vi "Com_Panel_Panel Fit Origin.vi"(8 "error in":errorcluster, 11 "VI Refnum In":refnum<vi>) -> (0 "error out":errorcluster, 3 "VI Refnum Out":refnum<vi>)   [LabVIEW 2016]
uses:
  <vilib>/Utility/miscctls.llb/LVPointTypeDef.ctl
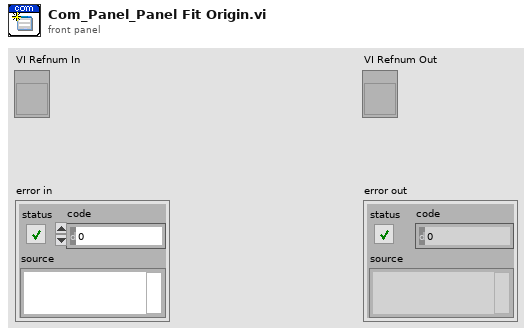
[diagram p1: front panel]
types:
  T1 = typedef "LVPointTypeDef.ctl" = cluster{"Horizontal":i16, "Vertical":i16}
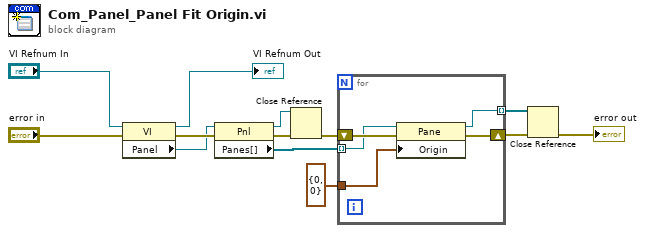
[diagram p0: block diagram]
diagram:
  n1 = property class="VI"(reference="VI Refnum In", error in="error in") -> (reference out=→"VI Refnum Out":refnum<vi>, error out=w13:errorcluster, "Panel"=w12:refnum<vi>)
  n2 = property class="Pnl"(reference=w12, error in=w13) -> (reference out=w10:refnum<vi>, error out=w9:errorcluster, "Panes[]"=w7:refnum<vi>[])
  n3 = Close Reference(reference=w10, error in (no error)=w9) -> (error out=w8:errorcluster)
  n4 = for {
    tunnel: w7 -> [w17] mode=indexing
    tunnel: T1 {"Horizontal"=0, "Vertical"=0} ("Origin") -> [w16]
    tunnel: [w14] -> w4 mode=indexing
    shift-right: [w15] -> w5
    shift-left: w8 -> [w18]
    n5 = property class="Pane"(reference=w17, error in=w18, "Origin"=w16) -> (reference out=w14:refnum<vi>, error out=w15:errorcluster)
  }
  n6 = Close Reference(reference=w4, error in (no error)=w5) -> (error out=→"error out":errorcluster)
